vi "ANC_MoveAbs.vi"(0 "Att DeviceHandle":u64, 1 "ourDLL":path, 2 "axis":u8(ring)=2 items=["1", "2", "3"], 3 "Target pos":dbl min=-500.0 max=3500.0 format="%#_7g", 5 "Att Error":errorcluster) -> (6 "deviceHandle out":u64, 7 "Out Position [µm | m°]":dbl, 8 "error out":errorcluster)   [LabVIEW 2019]
panel:
  in  "Att Pos Y 2":dbl min=-500.0 max=3500.0 format="%#_7g"
  in  "Att Pos Z":dbl min=-500.0 max=3500.0 format="%#_7g"
  in  "Att Pos Y":dbl min=-500.0 max=3500.0 format="%#_7g"
  in  "Att Pos X":dbl min=-500.0 max=3500.0 format="%#_7g"
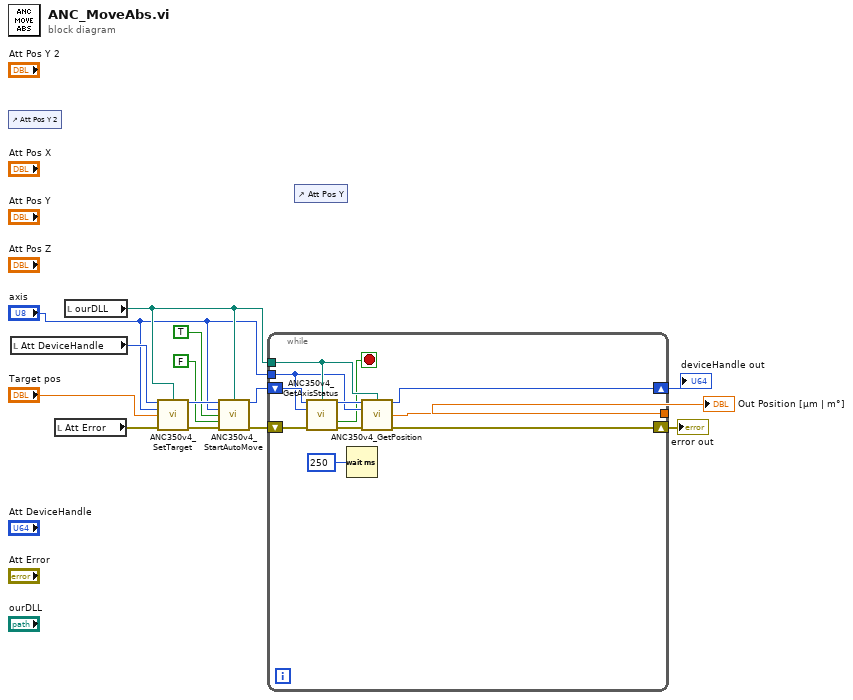
[diagram p0: block diagram]
diagram:
  n1 = control-ref of="Att Pos Y 2"() -> ()  [unwired: 1 out]
  n2 = local read "Att DeviceHandle"() -> (w7:u64)
  n3 = local read "Att Error"() -> (w8:errorcluster)
  n4 = local read "ourDLL"() -> (w13:path)
  n5 = call "ANC350v4_SetTarget.vi"("deviceHandle"=w7, "Path to *.DLL"=w13, "axis"="axis", "Target [µm | m°]"="Target pos", "error in"=w8) -> ("deviceHandle"=w9:u64, "error ANC350v4_setTarget"=w10:errorcluster)  [unwired: 8 in, 1 out]
  n6 = call "ANC350v4_StartAutoMove.vi"("deviceHandle"=w9, "Path to *.DLL"=w13, "axis"="axis", "Enable | Disable"=TRUE, "Relative | Absolute"=FALSE, "error in"=w10) -> ("deviceHandle out"=w11:u64, "error ANC350v4_StartAutoMove"=w12:errorcluster)  [unwired: 7 in, 1 out]
  n7 = while {
    tunnel: w13 -> [w20]
    shift-right: [w19] -> w3
    shift-left: w11 -> [w25]
    shift-right: [w18] -> w2
    shift-left: w12 -> [w24]
    tunnel: "axis" -> [w17]
    tunnel: [w15] -> w4
    stop <- w16 stop-if-true
    n8 = call "ANC350v4_GetAxisStatus.vi"("deviceHandle"=w25, "Path to *.DLL"=w20, "axis"=w17, "error in"=w24) -> ("deviceHandle"=w23:u64, "Target"=w16:bool, "error ANC350v4_getAxisStatus"=w22:errorcluster)  [unwired: 6 in, 3 out]
    n9 = Wait (ms)(milliseconds to wait=u32 250) -> ()  [unwired: 1 out]
    n10 = call "ANC350v4_GetPosition.vi"("deviceHandle"=w23, "Path to *.DLL"=w20, "axis"=w17, "error in"=w22) -> ("deviceHandle"=w19:u64, "Position [µm | m°]"=w15:dbl, "error ANC350v4_getPosition"=w18:errorcluster)  [unwired: 8 in, 1 out]
  }
  "Out Position [µm | m°]" <- w4
  "deviceHandle out" <- w3
  "error out" <- w2
  n11 = control-ref of="Att Pos Y"() -> ()  [unwired: 1 out]
